vi "Write Test status.vi"(7 "Send any changes now? (F)":bool, 8 "error in (no error)":errorcluster, 10 "Test status":string, 11 "Fiber Auto Collimation state data in":refnum<class "Fiber Auto Collimation state data.lvclass">) -> (0 "error out":errorcluster, 3 "Fiber Auto Collimation state data out":refnum<class "Fiber Auto Collimation state data.lvclass">)   [LabVIEW 2018, in "Fiber Auto Collimation state data.lvclass"]
doc: "Sets the \"Test status\" string. Basically, a very short description of what's happening to keep the user informed."
uses:
  Fiber Auto Collimation state data.lvclass
  Fiber Auto Collimation state data.lvclass/Fiber Auto Collimation state data.ctl
  Tracked state data.ctl
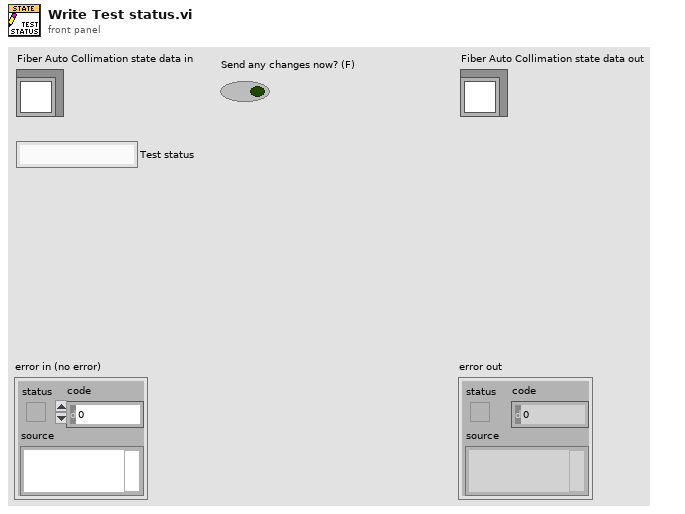
[diagram p1: front panel]
types:
  T1 = typedef "Fiber Auto Collimation state data.lvclass/Tracked state data.ctl" = enum16{"No update", "Permission level", "Username", "Test running", "DUT Serial", "Test status", "MOM Lot", "Loaded test recipe", "Model case running", "Station status", "BV data", "Defect Identify data", "Axis Position data", "Fiber Ass PN", "Operator", "RunTime", "VBAI", "Steps Cycle Time"}
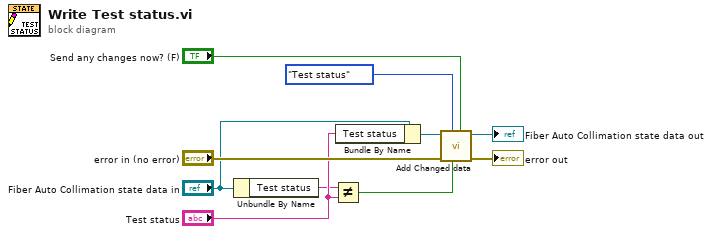
[diagram p0: block diagram]
diagram:
  n1 = Unbundle By Name("Fiber Auto Collimation state data in") -> ("Test status"=w2:string)
  n2 = Not Equal?(x=w2, y="Test status") -> (x != y?=w3:bool)
  n3 = Bundle By Name(cluster="Fiber Auto Collimation state data in", "Test status"="Test status") -> (w6:refnum<class "Fiber Auto Collimation state data.lvclass">)
  n4 = call "Add Changed data.vi"("Send any changes now? (F)"="Send any changes now? (F)", "Data changed?"=w3, "Data type"=Tracked_state_data."Test status", "error in (no error)"="error in (no error)", "Fiber Auto Collimation state data in"=w6) -> ("error out"=→"error out":errorcluster, "Fiber Auto Collimation state data out"=→"Fiber Auto Collimation state data out":refnum<class "Fiber Auto Collimation state data.lvclass">)  [unwired: 5 in]
